vi "GUI_PRD2000.vi"() -> ()   [LabVIEW 2013]
uses:
  Shared/GUI_Template/GUI_master/tcp_new_data_event.ctl
  Shared/GUI_Template/GUI_master/tcp new data cluster.ctl
panel:
  out "tcp data event":T1
  in  "Refresh Button":bool
  in  "Select device":string(combo)="BELLA_PDR2000"
  in  "stop":bool
  in  "pressure2::1":dbl=0.001 caption="Pressure 2" min=-100.0 max=500.0 format="%_4f"
  in  "pressure::1":dbl=0.001 caption="Pressure 1" min=-100.0 max=500.0 format="%_4p"
  in  "GUIdevice 1":string="BELLA_PDR2000"
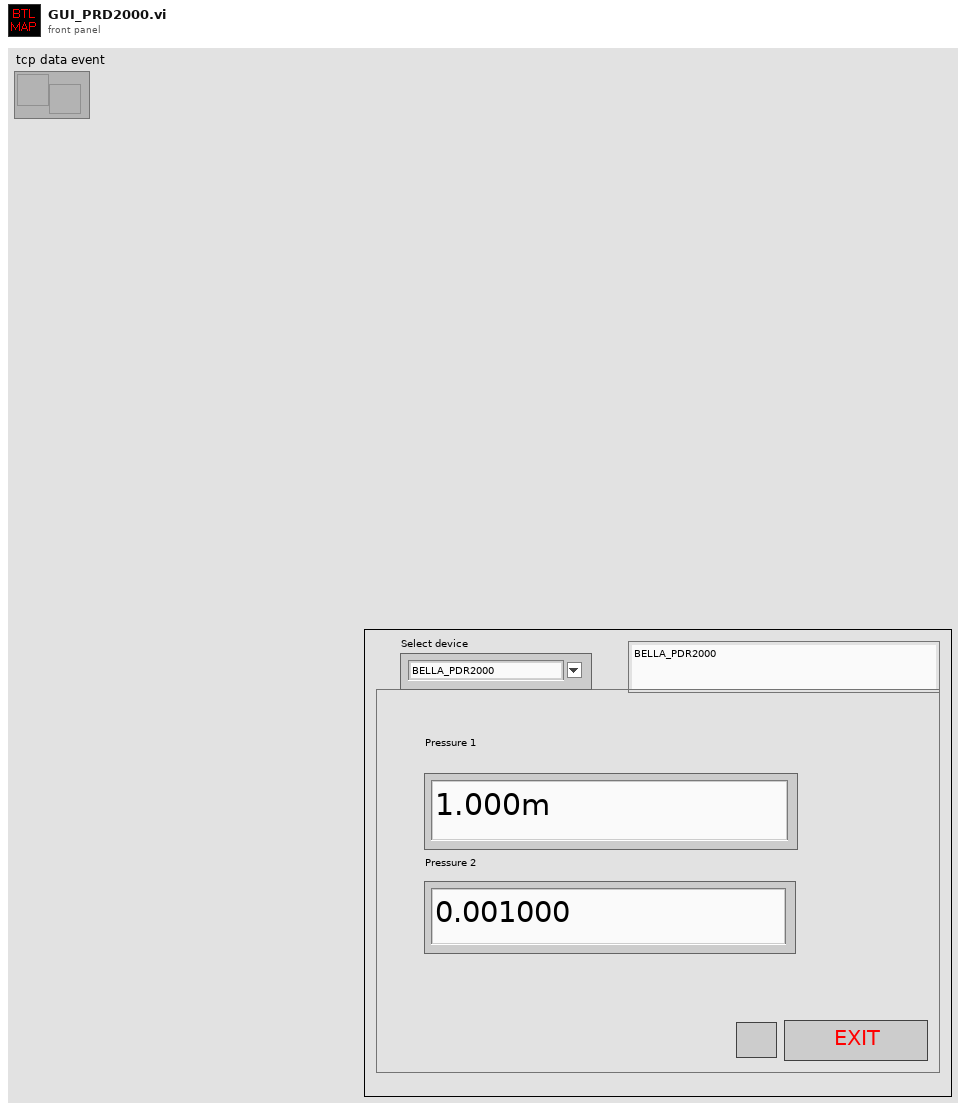
[diagram p1: front panel]
types:
  T1 = typedef "tcp_new_data_event.ctl" = refnum<user-event>
  T2 = enum32{"invalid app kind", "Development System", "Run Time System", "Student Edition", "Embedded LabVIEW", "Evaluation", "Custom"}
  T3 = typedef "tcp new data cluster.ctl" = cluster{"EventEnum":enum16{"new data", "connection status update"}, "Device name":string}
  T4 = enum32{"Invalid", "Standard", "Closed", "Hidden", "Minimized", "Maximized"}
  T5 = cluster{"Core":cluster{"Current VI Reference":refnum<vi>, "Close Panel on Exit?":bool}, "Your Boolean data":bool, "Your string data":string, "SuperGUI":cluster{"STOP queue":refnum<queue>, "SuperGUI ref":refnum<vi>}}
  T6 = cluster{"STOP queue":refnum<queue>, "SuperGUI ref":refnum<vi>}
  T7 = cluster{"Current VI Reference":refnum<vi>, "Close Panel on Exit?":bool}
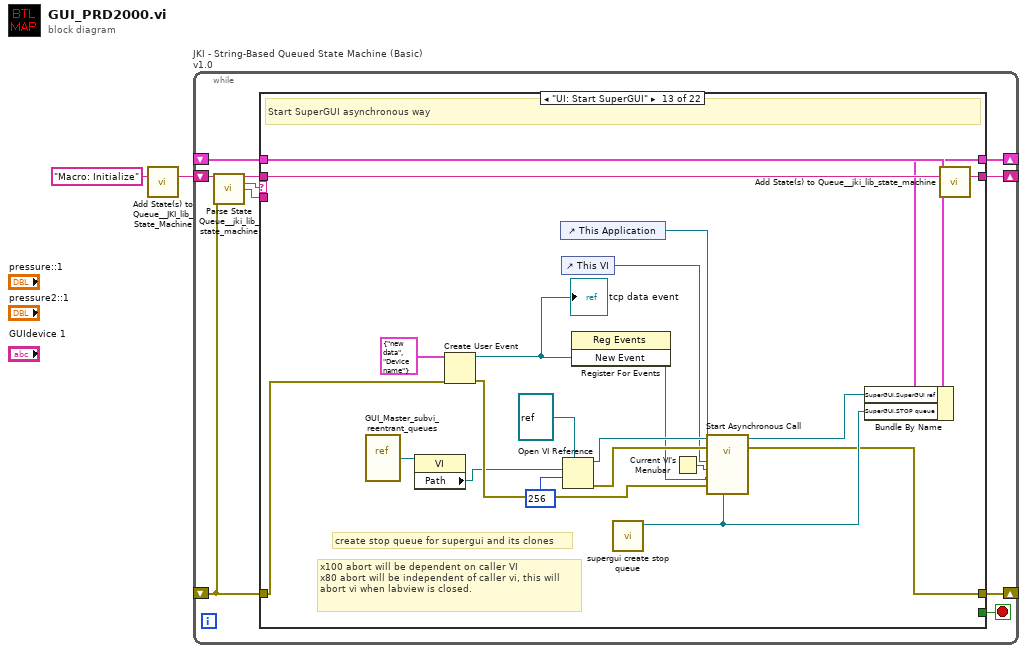
[diagram p0: block diagram]
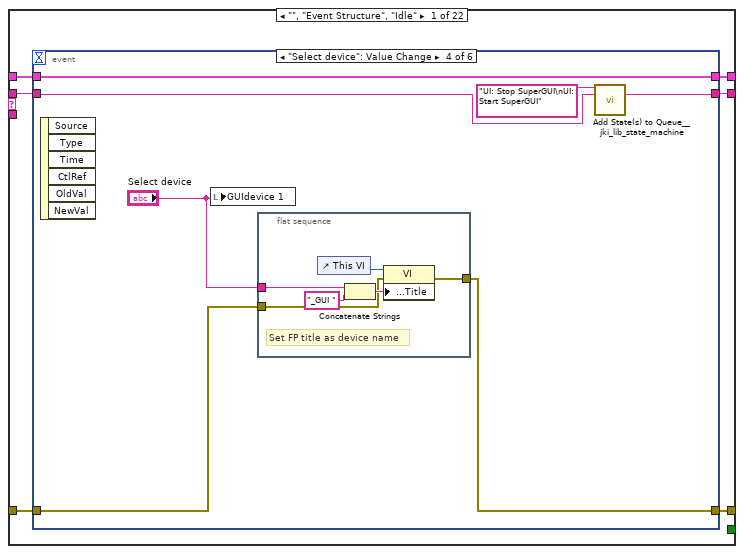
[diagram p2: hidden frame]
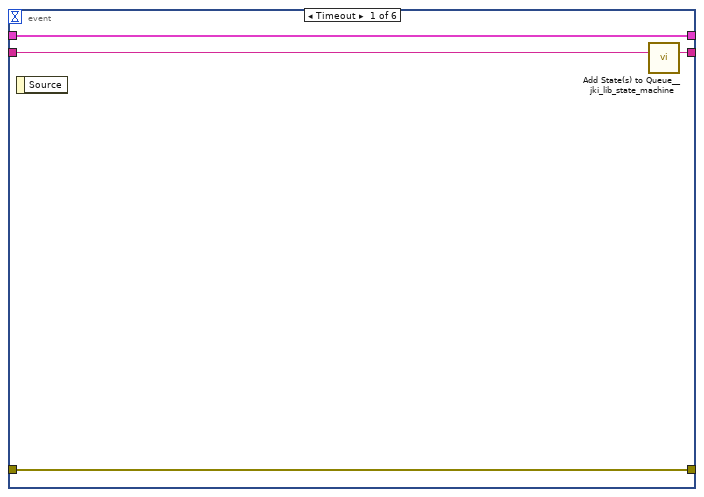
[diagram p3: hidden frame]
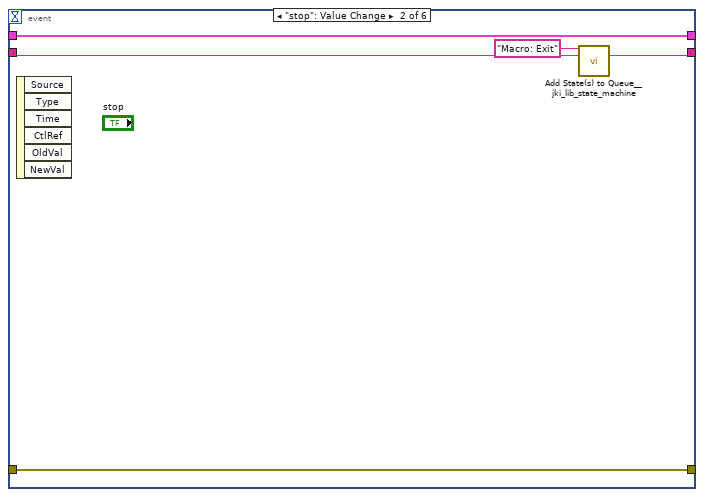
[diagram p4: hidden frame]
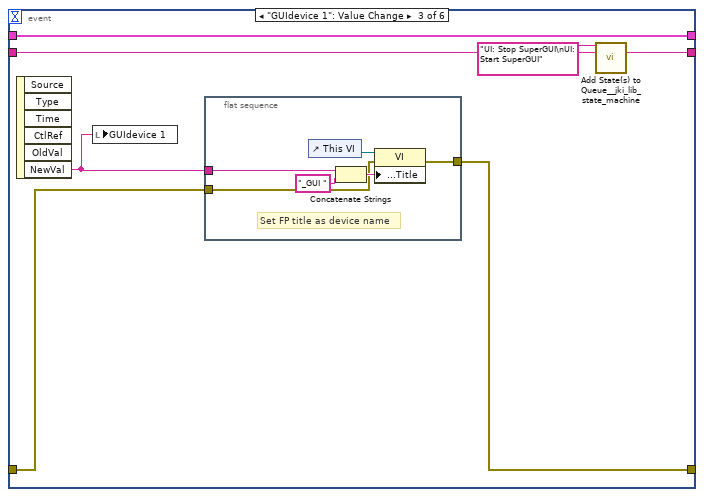
[diagram p5: hidden frame]
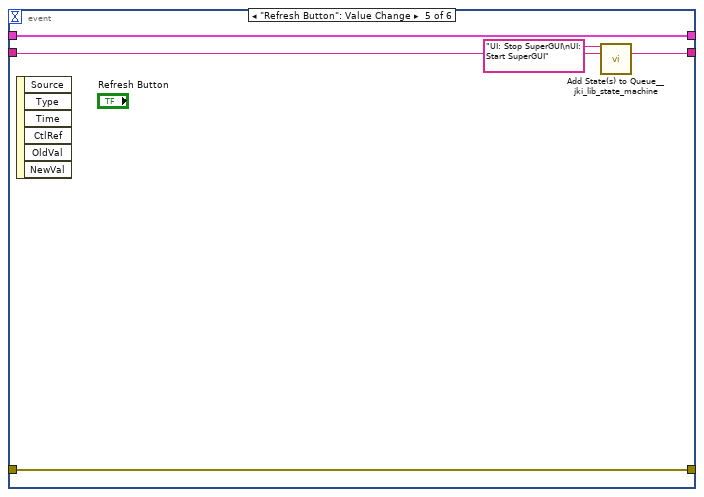
[diagram p6: hidden frame]
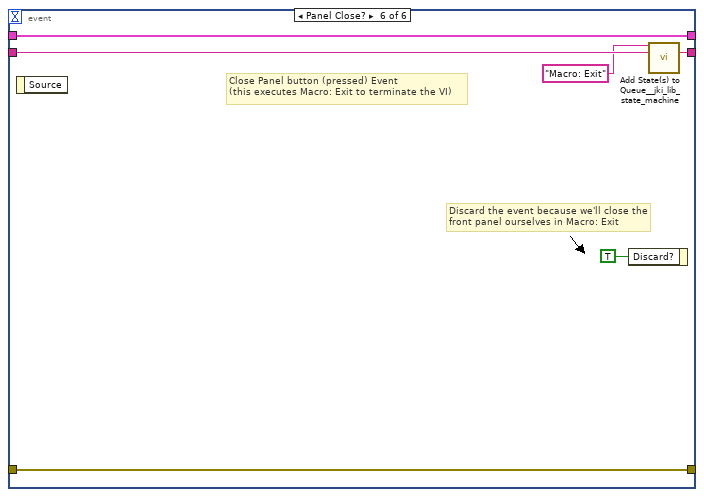
[diagram p7: hidden frame]
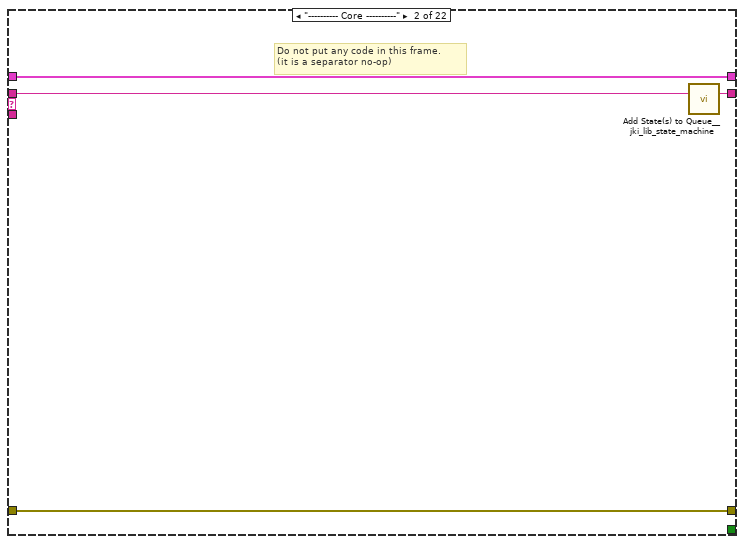
[diagram p8: hidden frame]
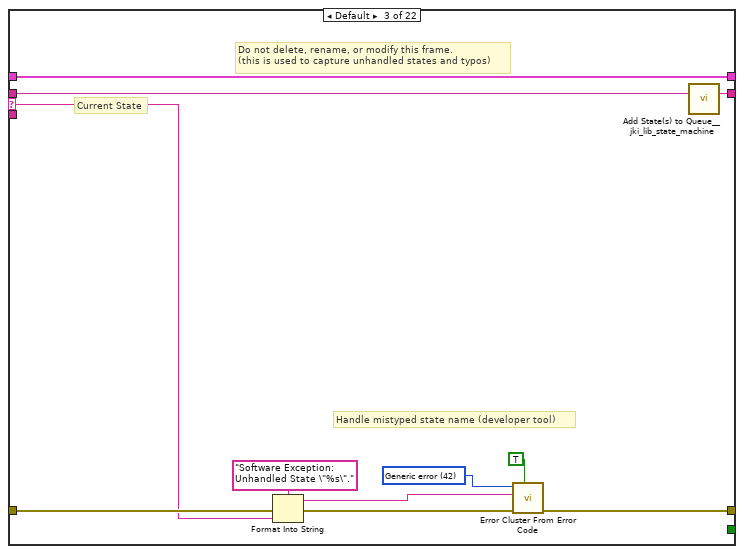
[diagram p9: hidden frame]
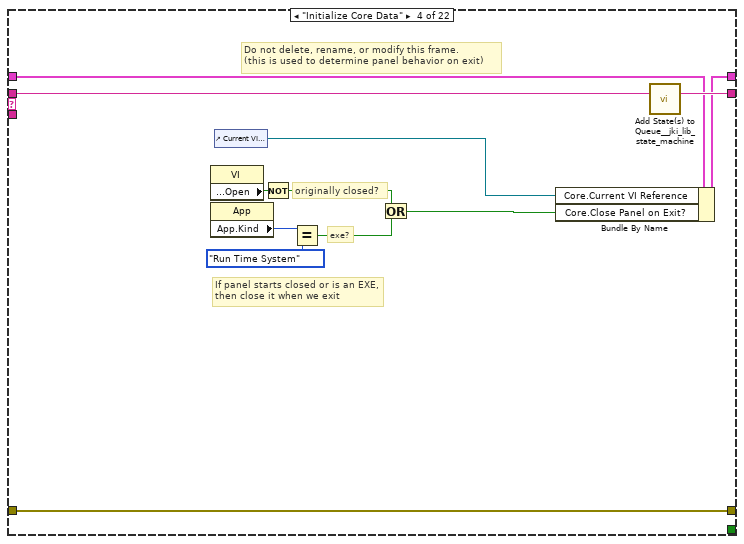
[diagram p10: hidden frame]
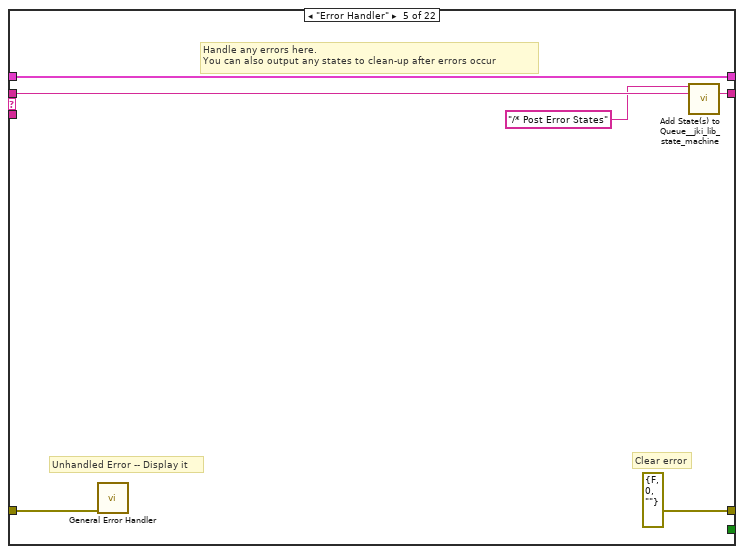
[diagram p11: hidden frame]
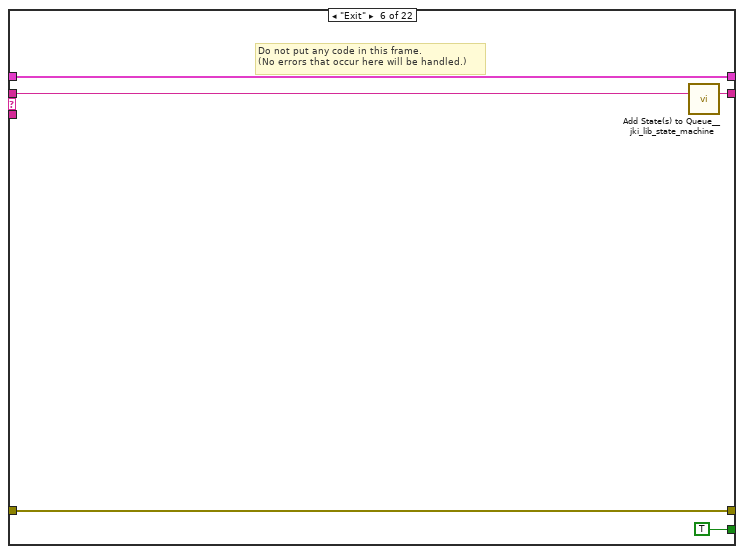
[diagram p12: hidden frame]
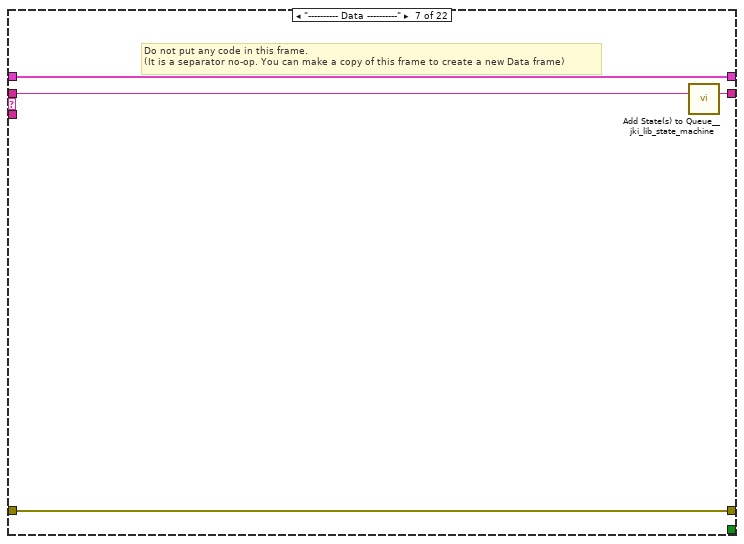
[diagram p13: hidden frame]
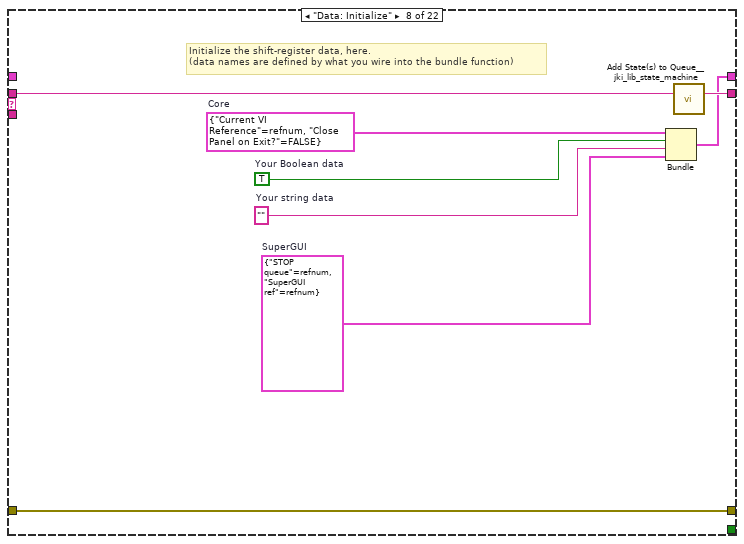
[diagram p14: hidden frame]
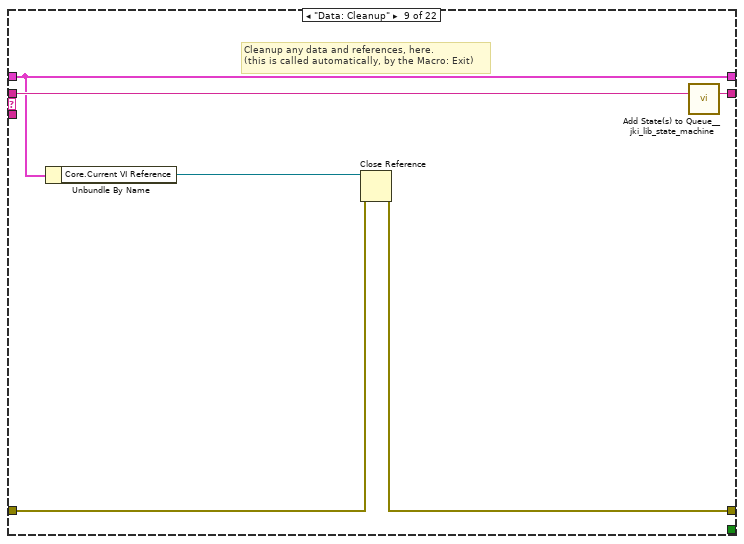
[diagram p15: hidden frame]
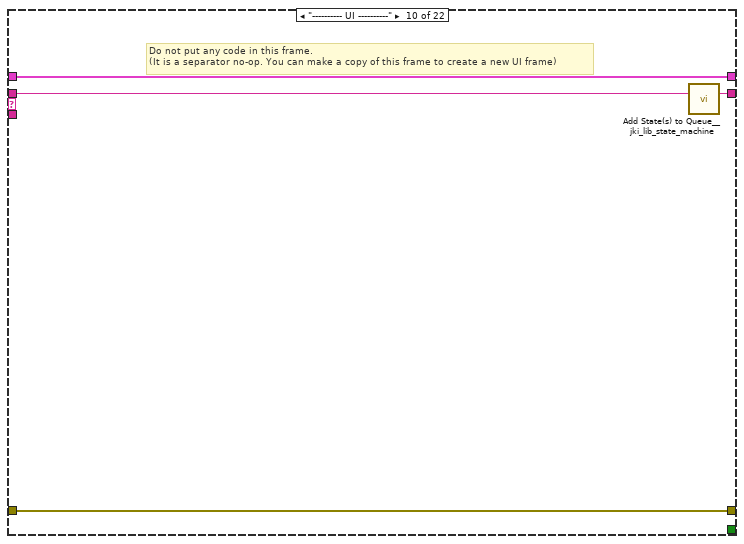
[diagram p16: hidden frame]
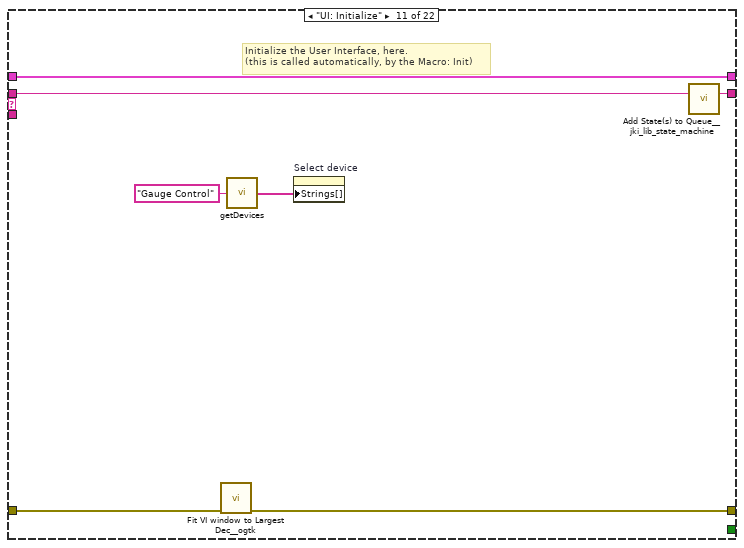
[diagram p17: hidden frame]
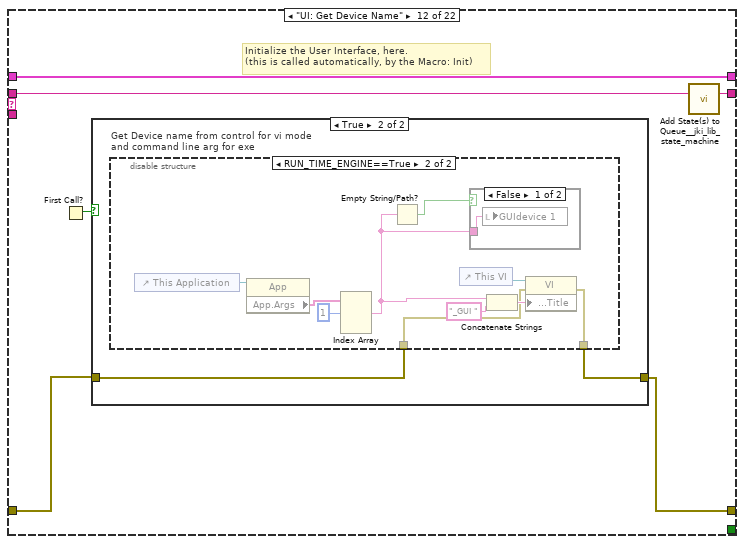
[diagram p18: hidden frame]
diagram:
  n1 = call <vilib>:"Add State(s) to Queue__JKI_lib_State_Machine.vi"("State(s) in (\"\")"="Macro: Initialize") -> ("States Out"=w1:string)  [unwired: 14 in]
  n2 = while "JKI - String-Based Queued State Machine (Basic) v1.0" {
    shift-right: [w5] -> _
    shift-left: _ -> [w4]
    shift-right: [w8] -> _
    shift-left: _ -> [w3]
    shift-right: [w7] -> _
    shift-left: w1 -> [w9]
    stop <- w6 stop-if-true
    n3 = call <vilib>:"Parse State Queue__jki_lib_state_machine.vi"("State Queue"=w9, "Error In (no error)"=w3) -> ("Remaining States"=w11:string, "Current State"=w12:string, "Arguments"=w10:string)  [unwired: 11 in]
    n4 = case shown="\"UI: Start SuperGUI\"" w12 {
      selector: w12 -> [_ _ w69 _ _ _ _ _ _ _ _ _ _ _ _ _ _ _ _ _ _ _]
      tunnel: w11 -> [w18 w68 w73 w91 w97 w102 w106 w114 w120 w124 w131 w137 w172 w180 w186 w197 w223 w228 w238 w242 w246 w250]
      tunnel: w10 -> [_ _ _ _ _ _ _ _ _ _ _ _ _ _ w181 w191 _ _ _ _ _ _]
      tunnel: w4 -> [w16 w65 w71 w82 w94 w100 w103 _ w115 w121 w129 w135 w163 w175 w184 w193 w220 w225 w235 w239 w243 w247]
      tunnel: [w15 w66 w75 w88 errorcluster {"status"=FALSE, "code"=0, "source"=""} ("error out") w99 w104 w111 w116 w122 w127 w132 w156 w173 w182 w194 w221 w226 w236 w240 w244 w248] -> w8
      tunnel: w3 -> [w14 w66 w74 w88 w93 w99 w104 w111 w117 w122 w128 w133 w157 w174 w183 w195 w221 w226 w236 w240 w244 w248]
      tunnel: [w17 w67 w72 w90 w96 w101 w105 w113 w119 w123 w130 w136 w171 w179 w185 w196 w222 w227 w237 w241 w245 w249] -> w7
      tunnel: [_ _ _ _ _ TRUE _ _ _ _ _ _ _ _ _ _ _ _ _ _ _ _] -> w6
      tunnel: [w13 w65 w71 w89 w94 w100 w103 w112 w115 w121 w129 w135 w162 w175 w184 w193 w220 w225 w235 w239 w243 w247] -> w5
      frame "", "Event Structure", "Idle" {
        n5 = event shown="[3] \"Select device\": Value Change" {
          selector: _ -> [_ _ _ _ _ _]
          dyn-events: _ -> [_ _ _ _ _ _]
          timeout: _ -> [_ _ _ _ _ _]
          tunnel: w18 -> [w22 w25 w31 w42 w56 w64]
          tunnel: [w21 w24 w30 w41 w55 w63] -> w17
          tunnel: w16 -> [w19 w27 w34 w47 w58 w61]
          tunnel: [w20 w26 w32 w44 w57 w62] -> w15
          tunnel: w14 -> [w20 w26 w33 w45 w57 w62]
          tunnel: [w19 w27 w34 w47 w58 w61] -> w13
          event Timeout {
            n6 = event-data() -> ()  [unwired: 1 in, 1 out]
            n7 = call <vilib>:"Add State(s) to Queue__jki_lib_state_machine.vi"("State(s) in (\"\")"=w22) -> ("States Out"=w21:string)  [unwired: 14 in]
          }
          event "stop": Value Change {
            n8 = event-data() -> ()  [unwired: 1 in, 6 out]
            n9 = call <vilib>:"Add State(s) to Queue__jki_lib_state_machine.vi"("State(s) in Front (\"\")"="Macro: Exit", "State(s) in (\"\")"=w25) -> ("States Out"=w24:string)  [unwired: 13 in]
          }
          event "GUIdevice 1": Value Change {
            n10 = event-data() -> ("NewVal"=w28:string)  [unwired: 1 in, 5 out]
            n11 = local write "GUIdevice 1"(w28) -> ()
            n12 = flat-sequence {
              tunnel: [w37] -> w32
              tunnel: w33 -> [w36]
              tunnel: w28 -> [w35]
              frame #0 {
                # "Set FP title as device name"
                n13 = control-ref of="This VI"() -> (w40:refnum<vi>)
                n14 = Concatenate Strings(w35, "_GUI ") -> (w39:string)
                n15 = property class="VI"(reference=w40, error in=w36, "Front Panel.Title"=w39) -> (error out=w37:errorcluster)  [unwired: 1 out]
              }
            }
            n16 = call <vilib>:"Add State(s) to Queue__jki_lib_state_machine.vi"("State(s) in Front (\"\")"="UI: Stop SuperGUI\nUI: Start SuperGUI", "State(s) in (\"\")"=w31) -> ("States Out"=w30:string)  [unwired: 13 in]
          }
          event "Select device": Value Change {
            n17 = event-data() -> ()  [unwired: 1 in, 6 out]
            n18 = local write "GUIdevice 1"("Select device") -> ()
            n19 = flat-sequence {
              tunnel: [w50] -> w44
              tunnel: w45 -> [w49]
              tunnel: "Select device" -> [w48]
              frame #0 {
                # "Set FP title as device name"
                n20 = control-ref of="This VI"() -> (w53:refnum<vi>)
                n21 = Concatenate Strings(w48, "_GUI ") -> (w52:string)
                n22 = property class="VI"(reference=w53, error in=w49, "Front Panel.Title"=w52) -> (error out=w50:errorcluster)  [unwired: 1 out]
              }
            }
            n23 = call <vilib>:"Add State(s) to Queue__jki_lib_state_machine.vi"("State(s) in Front (\"\")"="UI: Stop SuperGUI\nUI: Start SuperGUI", "State(s) in (\"\")"=w42) -> ("States Out"=w41:string)  [unwired: 13 in]
          }
          event "Refresh Button": Value Change {
            n24 = event-data() -> ()  [unwired: 1 in, 6 out]
            n25 = call <vilib>:"Add State(s) to Queue__jki_lib_state_machine.vi"("State(s) in Front (\"\")"="UI: Stop SuperGUI\nUI: Start SuperGUI", "State(s) in (\"\")"=w56) -> ("States Out"=w55:string)  [unwired: 13 in]
          }
          event Panel Close? {
            # "Discard the event because we'll close the front panel ourselves in Macro: Exit"
            # "Close Panel button (pressed) Event\n(this executes Macro: Exit to terminate the VI)"
            n26 = event-data() -> ()  [unwired: 1 in, 1 out]
            n27 = event-data("Discard?"=TRUE) -> ()  [unwired: 1 in, 1 out]
            n28 = call <vilib>:"Add State(s) to Queue__jki_lib_state_machine.vi"("State(s) in Front (\"\")"="Macro: Exit", "State(s) in (\"\")"=w64) -> ("States Out"=w63:string)  [unwired: 13 in]
          }
        }
      }
      frame "---------- Core ----------" {
        # "Do not put any code in this frame.\n(it is a separator no-op)"
        n29 = call <vilib>:"Add State(s) to Queue__jki_lib_state_machine.vi"("State(s) in (\"\")"=w68) -> ("States Out"=w67:string)  [unwired: 14 in]
      }
      frame Default {
        w78 = 42 items=["No error", "Argument error", "Memory is full", "Out of zone", "End of file", "File already open", "Generic file I/O error", "File not found", "File permission error", "Disk is full", "Duplicate path", "Too many files open", "System feature not enabled", "Resource file not found", "Cannot add resource", "Resource not found", "Image not found", "Image memory error", "Pen does not exist", "Config type invalid", "Config token not found", "Config parse error", "Config memory error", "Bad external code format", "Bad external code offset", "External code not present", "Null window", "Destroy window error", "Null menu", "Print aborted", "Bad print record", "Print driver error", "Windows error during printing", "Memory error during printing", "Print dialog error", "Generic print error", "Invalid device refnum", "Device not found", "Device parameter error", "Device unit error", "Cannot open device", "Device call aborted", "Generic error", "Cancelled by user", "Object ID too low", "Object ID too high", "Object not in heap", "Unknown heap", "Unknown object (invalid DefProc)", "Unknown object (DefProc not in table)", "Message out of range", "Invalid (null) method", "Unknown message", "Manager call not supported", "Bad address", "Network operation in progress", "Network operation timed out", "Connection is busy", "Network attribute not supported", "Network error", "Address in use", "System out of memory", "Connection aborted", "Connection refused", "Not connected", "Already connected", "Connection closed", "Initialization error (interapplication manager)", "Bad occurrence", "Wait on unbound occurrence handler", "Occurrence queue overflow", "Datalog type conflict", "Unused", "Unrecognized type (interapplication manager)", "Memory corrupt", "Failed to make temporary DLL", "Old CIN version", "Drag socket not found", "Failed to load drop-object", "Failed to register OLE object", "Failed to release OLE object", "Format specifier type mismatch", "Unknown format specifier", "Too few format specifiers", "Too many format specifiers", "Scan failed", "Newer CIN version", "Error converting to variant", "Runtime menu error", "Password tampered", "Variant attribute not found", "Incompatible variant data type", "Event data is not available", "Event Store is not present", "Occurrence is not found", "Event Queue is not created", "Event info is not available", "Refnum passed is NULL", "Error retrieving Class GUID", "Error retrieving CoClass GUID", "Error retrieving TypeLib GUID.", "Bad built application magic bytes.", "Specific driver is different from the specific driver associated with the Logical Name.", "There is no session opened to the class driver.", "Max Error", "MAX - Error with config objects", "MAX - Error loading configuration", "MAX - Group not supported"]
        # "Current State"
        # "Do not delete, rename, or modify this frame.\n(this is used to capture unhandled states and typos)"
        # "Handle mistyped state name (developer tool)"
        n30 = Format Into String(format string="Software Exception: Unhandled State \"%s\"." ("message"), error in=w74, w69) -> (resulting string=w77:string, error out=w76:errorcluster)  [unwired: 1 in]
        n31 = call <vilib>:"Error Cluster From Error Code.vi"("show call chain? (False)"=TRUE, "error in (no error)"=w76, "error message (\"\")"=w77, "error code (0)"=w78) -> ("error out"=w75:errorcluster)  [unwired: 5 in]
        n32 = call <vilib>:"Add State(s) to Queue__jki_lib_state_machine.vi"("State(s) in (\"\")"=w73) -> ("States Out"=w72:string)  [unwired: 14 in]
      }
      frame "Initialize Core Data" {
        # "Do not delete, rename, or modify this frame.\n(this is used to determine panel behavior on exit)"
        # "originally closed?"
        # "exe?"
        # "If panel starts closed or is an EXE, then close it when we exit"
        n33 = property class="VI"() -> ("Front Panel.Open"=w87:bool)  [unwired: 2 in, 2 out]
        n34 = property class="App"() -> ("App.Kind"=w86:T2)  [unwired: 2 in, 2 out]
        n35 = control-ref of="Current VI Reference"() -> (w80:refnum<vi>)
        n36 = Not(x=w87) -> (.not. x?=w84:bool)
        n37 = Equal?(x=w86, y=T2."Run Time System" ("Application:Kind")) -> (x = y?=w83:bool)
        n38 = Or(x=w84, y=w83) -> (x .or. y?=w81:bool)
        n39 = Bundle By Name(cluster=w82, "Core.Current VI Reference"=w80, "Core.Close Panel on Exit?"=w81) -> (w89:T5)
        n40 = call <vilib>:"Add State(s) to Queue__jki_lib_state_machine.vi"("State(s) in (\"\")"=w91) -> ("States Out"=w90:string)  [unwired: 14 in]
      }
      frame "Error Handler" {
        # "Unhandled Error -- Display it"
        # "Handle any errors here.\nYou can also output any states to clean-up after errors occur"
        # "Clear error"
        n41 = call <vilib>:"General Error Handler.vi"("error in (no error)"=w93) -> ()  [unwired: 10 in, 5 out]
        n42 = call <vilib>:"Add State(s) to Queue__jki_lib_state_machine.vi"("State(s) in Front (\"\")"="/* Post Error States", "State(s) in (\"\")"=w97) -> ("States Out"=w96:string)  [unwired: 13 in]
      }
      frame "Exit" {
        # "Do not put any code in this frame.\n(No errors that occur here will be handled.)"
        n43 = call <vilib>:"Add State(s) to Queue__jki_lib_state_machine.vi"("State(s) in (\"\")"=w102) -> ("States Out"=w101:string)  [unwired: 14 in]
      }
      frame "---------- Data ----------" {
        # "Do not put any code in this frame.\n(It is a separator no-op. You can make a copy of this frame to create a new Data frame)"
        n44 = call <vilib>:"Add State(s) to Queue__jki_lib_state_machine.vi"("State(s) in (\"\")"=w106) -> ("States Out"=w105:string)  [unwired: 14 in]
      }
      frame "Data: Initialize" {
        w107 = T6 {"STOP queue"=refnum, "SuperGUI ref"=refnum}  # SuperGUI
        w108 = T7 {"Current VI Reference"=refnum, "Close Panel on Exit?"=FALSE}  # Core
        w110 = TRUE  # Your Boolean data
        w109 = ""  # Your string data
        # "Initialize the shift-register data, here.\n(data names are defined by what you wire into the bundle function)"
        n45 = Bundle("Core"=w108, "Your Boolean data"=w110, "Your string data"=w109, "SuperGUI"=w107) -> (w112:T5)  [unwired: 1 in]
        n46 = call <vilib>:"Add State(s) to Queue__jki_lib_state_machine.vi"("State(s) in (\"\")"=w114) -> ("States Out"=w113:string)  [unwired: 14 in]
      }
      frame "Data: Cleanup" {
        # "Cleanup any data and references, here.\n(this is called automatically, by the Macro: Exit)"
        n47 = Unbundle By Name(w115) -> ("Core.Current VI Reference"=w118:refnum<vi>)
        n48 = Close Reference(reference=w118, error in (no error)=w117) -> (error out=w116:errorcluster)
        n49 = call <vilib>:"Add State(s) to Queue__jki_lib_state_machine.vi"("State(s) in (\"\")"=w120) -> ("States Out"=w119:string)  [unwired: 14 in]
      }
      frame "---------- UI ----------" {
        # "Do not put any code in this frame.\n(It is a separator no-op. You can make a copy of this frame to create a new UI frame)"
        n50 = call <vilib>:"Add State(s) to Queue__jki_lib_state_machine.vi"("State(s) in (\"\")"=w124) -> ("States Out"=w123:string)  [unwired: 14 in]
      }
      frame "UI: Initialize" {
        # "Initialize the User Interface, here.\n(this is called automatically, by the Macro: Init)"
        n51 = call <userlib>:"Fit VI window to Largest Dec__ogtk.vi"("error in (no error)"=w128) -> ("error out"=w127:errorcluster)  [unwired: 5 in, 1 out]
        n52 = call "getDevices.vi"("Device Class"="Gauge Control") -> ("All Devices"=w125:string[])
        n53 = property on="Select device" class="CmbBox"("Strings[]"=w125) -> ()  [unwired: 2 in, 2 out]
        n54 = call <vilib>:"Add State(s) to Queue__jki_lib_state_machine.vi"("State(s) in (\"\")"=w131) -> ("States Out"=w130:string)  [unwired: 14 in]
      }
      frame "UI: Get Device Name" {
        # "Initialize the User Interface, here.\n(this is called automatically, by the Macro: Init)"
        n55 = First Call?() -> (First Call?: T/F=w134:bool)
        n56 = case shown="True" w134 {
          tunnel: w133 -> [w138 w140]
          tunnel: [w138 w139] -> w132
          frame False {
          }
          frame True {
            n57 = disable-structure "Get Device name from control for vi mode\nand command line arg for exe" shown="RUN_TIME_ENGINE==True" {
              disable-tunnel: w140 -> [w141 w143]
              disable-tunnel: [w141 w142] -> w139
              frame condition #0 (active) {
              }
              frame condition #1 {
                n58 = control-ref of="This Application"() -> (w151:refnum<vi>)
                n59 = property class="App"(reference=w151) -> ("App.Args"=w150:string[])  [unwired: 1 in, 2 out]
                n60 = Index Array(array=w150, index #1=1 ("index")) -> (element #1=w144:string)  [unwired: 2 in, 2 out]
                n61 = Empty String/Path?(string/path=w144) -> (empty?=w148:bool)
                n62 = control-ref of="This VI"() -> (w147:refnum<vi>)
                n63 = case shown="False" w148 {
                  tunnel: w144 -> [w152 _]
                  frame False {
                    n64 = local write "GUIdevice 1"(w152) -> ()
                  }
                  frame True {
                  }
                }
                n65 = Concatenate Strings(w144, "_GUI ") -> (w146:string)
                n66 = property class="VI"(reference=w147, error in=w143, "Front Panel.Title"=w146) -> (error out=w142:errorcluster)  [unwired: 1 out]
              }
            }
          }
        }
        n67 = call <vilib>:"Add State(s) to Queue__jki_lib_state_machine.vi"("State(s) in (\"\")"=w137) -> ("States Out"=w136:string)  [unwired: 14 in]
      }
      frame "UI: Start SuperGUI" {
        # "create stop queue for supergui and its clones"
        # "x100 abort will be dependent on caller VI\nx80 abort will be independent of caller vi, this will abort vi when labview is closed."
        # "Start SuperGUI asynchronous way"
        n68 = vi-ref "GUI_Master_subvi_reentrant_queues.vi"() -> (w155:refnum<vi>)
        n69 = property class="VI"(reference=w155) -> ("Path"=w154:path)  [unwired: 1 in, 2 out]
        n70 = Create User Event(user event datatype=T3 {"EventEnum"=enum."new data", "Device name"="Device name"} ("New Event"), error in=w157) -> (user event=w158:refnum<user-event>, error out=w164:errorcluster)
        "tcp data event" <- w158
        n71 = control-ref of="This Application"() -> (w161:refnum<vi>)
        n72 = control-ref of="This VI"() -> (w160:refnum<vi>)
        n73 = Open VI Reference(type specifier VI Refnum (for type only)=refnum<vi> refnum, vi path=w154, options=256) -> (vi reference=w170:refnum<vi>, error out=w169:errorcluster)  [unwired: 3 in]
        n74 = register-events(w158) -> ()  [unwired: 2 in, 2 out]
        n75 = call "supergui create stop queue.vi"() -> ("STOP Queue out"=w166:refnum<queue>)  [unwired: 11 in]
        n76 = Current VI's Menubar() -> (w159:refnum<k9>)
        n77 = call-by-ref "Start Asynchronous Call"(reference=w170, error in=w169, "STOP Queue in"=w166, "This Application"=w161, 8:"error in (no error)"=w164, "tcp data event"=w158, "Caller menu reference"=w159, "Caller VI ref"=w160) -> (reference out=w153:refnum<vi>, error out=w156:errorcluster)  [unwired: 5 in, 1 out]
        n78 = Bundle By Name(cluster=w163, "SuperGUI.SuperGUI ref"=w153, "SuperGUI.STOP queue"=w166) -> (w162:T5)
        n79 = call <vilib>:"Add State(s) to Queue__jki_lib_state_machine.vi"("State(s) in (\"\")"=w172) -> ("States Out"=w171:string)  [unwired: 14 in]
      }
      frame "UI: Stop SuperGUI" {
        # "Stop Supergui Clone and wait until it exit properly"
        n80 = Unbundle By Name(w175) -> ("SuperGUI.SuperGUI ref"=w177:refnum<vi>, "SuperGUI.STOP queue"=w176:refnum<queue>)
        n81 = Release Queue(queue=w176, error in (no error)=w174) -> (error out=w178:errorcluster)  [unwired: 1 in, 2 out]
        n82 = call-by-ref "Wait On Asynchronous Call"(reference=w177, error in=w178) -> ("error out"=w173:errorcluster)  [unwired: 11 in, 2 out]
        n83 = call <vilib>:"Add State(s) to Queue__jki_lib_state_machine.vi"("State(s) in (\"\")"=w180) -> ("States Out"=w179:string)  [unwired: 14 in]
      }
      frame "UI: Cursor Set" {
        # "Argument"
        # "Set and Unset Cursor Busy.\n(Usage: \"UI: Cursor Set >> Busy|Idle\")"
        n84 = case shown="\"Idle\", Default" w181 {
          tunnel: w183 -> [w188 w190]
          tunnel: [w187 w189] -> w182
          frame "Idle", Default {
            n85 = call <vilib>:"Unset Busy.vi"("error in (no error)"=w188) -> ("error out"=w187:errorcluster)  [unwired: 10 in]
          }
          frame "Busy" {
            n86 = call <vilib>:"Set Busy.vi"("error in (no error)"=w190) -> ("error out"=w189:errorcluster)  [unwired: 9 in, 1 out]
          }
        }
        n87 = call <vilib>:"Add State(s) to Queue__jki_lib_state_machine.vi"("State(s) in (\"\")"=w186) -> ("States Out"=w185:string)  [unwired: 14 in]
      }
      frame "UI: Front Panel State" {
        # "Argument"
        # "Set Front Panel Open or Closed\n(Usage: \"UI: Front Panel State >> Open|Close\")"
        n88 = Unbundle By Name(w193) -> ("Core.Current VI Reference"=w192:refnum<vi>)
        n89 = case shown="\"Open\", Default" w191 {
          tunnel: w195 -> [w201 w214]
          tunnel: [w203 w215] -> w194
          tunnel: w192 -> [w202 w212]
          frame "Open", Default {
            n90 = property class="VI"(reference=w202, error in=w201) -> (reference out=w199:refnum<vi>, error out=w200:errorcluster, "Front Panel.Open"=w198:bool)
            n91 = case shown="False" w198 {
              tunnel: [w206 w209] -> w203
              tunnel: w200 -> [w205 w209]
              tunnel: w199 -> [w204 _]
              frame False {
                n92 = invoke class="VI" method="FP.Open"(reference=w204, error in=w205, "Activate"=TRUE, "State"=T4."Standard") -> (error out=w206:errorcluster)  [unwired: 1 in, 4 out]
              }
              frame True {
              }
            }
          }
          frame "Close" {
            n93 = property class="VI"(reference=w212, error in=w214) -> (reference out=w211:refnum<vi>, error out=w213:errorcluster, "Front Panel.Open"=w210:bool)
            n94 = case shown="True" w210 {
              tunnel: [w216 w219] -> w215
              tunnel: w213 -> [w216 w218]
              tunnel: w211 -> [_ w217]
              frame False {
              }
              frame True {
                n95 = invoke class="VI" method="FP.Close"(reference=w217, error in=w218) -> (error out=w219:errorcluster)  [unwired: 1 in, 2 out]
              }
            }
          }
        }
        n96 = call <vilib>:"Add State(s) to Queue__jki_lib_state_machine.vi"("State(s) in (\"\")"=w197) -> ("States Out"=w196:string)  [unwired: 14 in]
      }
      frame "---------- Macro ----------" {
        # "Do not put any code in this frame.\n(It is a separator no-op. You can make a copy of this frame to create a new Macro frame)"
        n97 = call <vilib>:"Add State(s) to Queue__jki_lib_state_machine.vi"("State(s) in (\"\")"=w223) -> ("States Out"=w222:string)  [unwired: 14 in]
      }
      frame "Macro: Initialize" {
        # "Initialization Macro\n(This is called once, when the VI starts)"
        n98 = call <vilib>:"Add State(s) to Queue__jki_lib_state_machine.vi"("State(s) in Front (\"\")"="Data: Initialize\nInitialize Core Data\nUI: Initialize\nUI: Get Device Name\nUI: Start SuperGUI\nUI: Front Panel State >> Open", "State(s) in (\"\")"=w228) -> ("States Out"=w227:string)  [unwired: 13 in]
      }
      frame "Macro: Exit" {
        # "Exit Macro\n(This is called once, when the VI exits)"
        n99 = Unbundle By Name(w235) -> ("Core.Close Panel on Exit?"=w234:bool)
        n100 = Select(t="UI: Front Panel State >> Close", s=w234, f="") -> (s? t:f=w231:string)
        n101 = call <vilib>:"Add State(s) to Queue__jki_lib_state_machine.vi"("State(s) in (\"\")"=w231, "State(s) at Back (\"\")"="Data: Cleanup\nExit") -> ("States Out"=w229:string)  [unwired: 13 in]
        n102 = call <vilib>:"Add State(s) to Queue__jki_lib_state_machine.vi"("State(s) in Front (\"\")"=w229, "State(s) in (\"\")"=w238) -> ("States Out"=w237:string)  [unwired: 13 in]
      }
      frame "---------- New Category ----------" {
        # "Template Separator\n(You can make a copy of, or modify, this frame)"
        n103 = call <vilib>:"Add State(s) to Queue__jki_lib_state_machine.vi"("State(s) in (\"\")"=w242) -> ("States Out"=w241:string)  [unwired: 14 in]
      }
      frame "New Category: 1" {
        # "Your code here.\n(You can make a copy of, or modify, this frame)"
        n104 = call <vilib>:"Add State(s) to Queue__jki_lib_state_machine.vi"("State(s) in (\"\")"=w246) -> ("States Out"=w245:string)  [unwired: 14 in]
      }
      frame "New Category: 2" {
        # "Your code here.\n(You can make a copy of, or modify, this frame)"
        n105 = call <vilib>:"Add State(s) to Queue__jki_lib_state_machine.vi"("State(s) in (\"\")"=w250) -> ("States Out"=w249:string)  [unwired: 14 in]
      }
    }
  }
